vi "Do.vi"(8 "error in (no error)":errorcluster, 10 "Actor in":refnum<class "Actor.lvclass">, 11 "Lock Publication Msg":refnum<class "Lock Publication Msg.lvclass">) -> (0 "error out":errorcluster, 2 "Actor out":refnum<class "Actor.lvclass">)   [LabVIEW 2017, in "IMediator.lvlib" / "Lock Publication Msg.lvclass"]
doc: "This VI delivers the message to the actor by calling the appropriate method(s) on the actor.\n\n<License>\nCopyright © 2017 Composed Systems, LLC | All rights reserved\nwww.composed.io\n\nAuthor: Ethan Stern <ethan.stern@composed.io>\n\nThis software is provided \"AS IS\" WITHOUT WARRANTIES, either express or implied, AND IS FOR EDUCATIONAL PURPOSES ONLY.\n</License>"
uses:
  Lock Publication Msg.lvclass
  <vilib>/ActorFramework/Actor/Actor.lvclass
  IMediator/IMediator.lvclass
  C:/Program Files (x86)/National Instruments/LabVIEW 2017/vi.lib/ActorFramework/Actor/Actor.lvclass
  Lock Publication Msg.lvclass/Lock Publication Msg.ctl
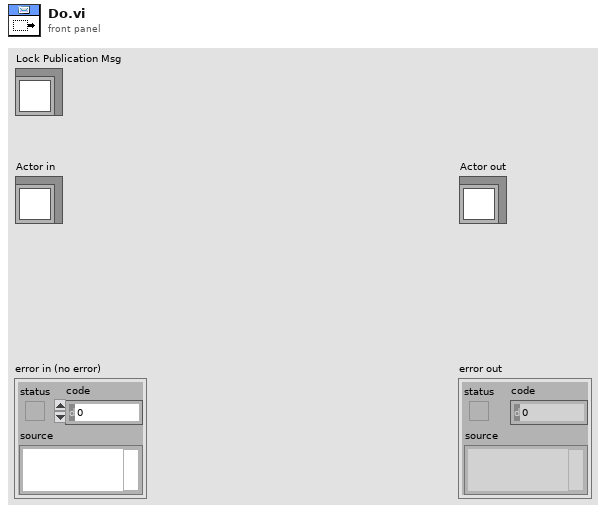
[diagram p1: front panel]
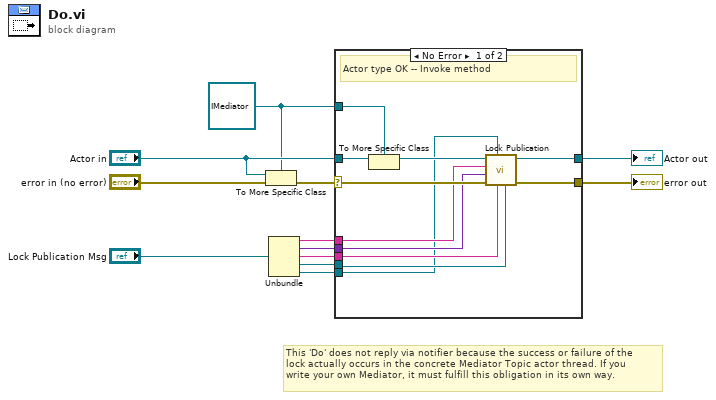
[diagram p0: block diagram]
diagram:
  w6 = refnum<class "IMediator.lvclass"> refnum ("Actor in")
  # "This 'Do' does not reply via notifier because the success or failure of the\nlock actually occurs in the concrete Mediator Topic actor thread. If you\nwrite your own Mediator, it must fulfill this obligation in its own way."
  n1 = To More Specific Class(target class=w6, reference="Actor in", error in="error in (no error)") -> (error out=w10:errorcluster)  [unwired: 1 out]
  n2 = Unbundle("Lock Publication Msg") -> (w5:string, w4:variant, w3:string, w2:refnum<class "ITransport.lvclass">, w1:refnum<class "IPublicationPolicy.lvclass">)
  n3 = case shown="No Error" w10 {
    selector: w10 -> [w21 w25]
    tunnel: [w23 w25] -> w9
    tunnel: [w22 w24] -> w8
    tunnel: "Actor in" -> [w20 w24]
    tunnel: w6 -> [w19 _]
    tunnel: w5 -> [w17 _]
    tunnel: w4 -> [w18 _]
    tunnel: w3 -> [w15 _]
    tunnel: w2 -> [w14 _]
    tunnel: w1 -> [w13 _]
    frame No Error {
      # "Actor type OK -- Invoke method"
      n4 = To More Specific Class(target class=w19, reference=w20) -> (specific class reference=w16:refnum<class "IMediator.lvclass">)  [unwired: 1 in, 1 out]
      n5 = call-dynamic "Lock Publication.vi"("Return Error Transport"=w14, "Publisher ID"=w15, "PublicationPolicy"=w13, "error in (no error)"=w21, "Datum Type"=w18, "Datum Name"=w17, "IMediator In"=w16) -> ("error out"=w23:errorcluster, "IMediator Out"=w22:refnum<class "IMediator.lvclass">)  [unwired: 3 in]
    }
    frame Error {
      # "If type check fails, pass the\noriginal object out again."
      # "Invalid Actor type"
    }
  }
  "error out" <- w9
  "Actor out" <- w8
